vi "Intensity.vi"(8 "error in (no error)":errorcluster, 10 "Image in":T2(plugin-control), 11 "Intensity Limit":string[][](array[string])) -> (0 "error out":errorcluster, 2 "Image out":T2(plugin-control), 3 "Intensity":T1(array[cluster]))   [LabVIEW 2020]
uses:
  <vilib>/vision/NI_Vision_Development_Module.lvlib
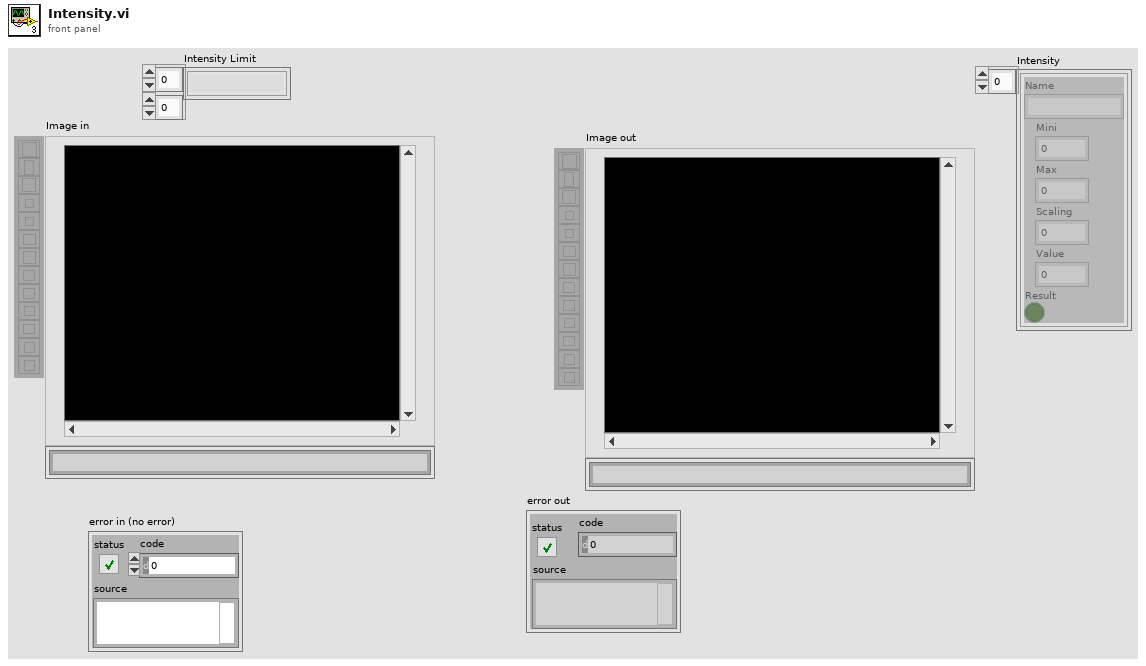
[diagram p1: front panel]
types:
  T1 = cluster{"Name":string, "Mini":dbl, "Max":dbl, "Scaling ":dbl, "Value ":dbl, "Result":bool}[]
  T2 = typedef "IMAQ Image.ctl" = refnum<image>
  T3 = cluster{"Name":string, "Mini":dbl, "Max":dbl, "Scaling ":dbl, "Value ":dbl, "Result":bool}
  T4 = cluster{"Global Rectangle":i32[], "Contours":cluster{"Contour Type":u32, "ROI Type":u32, "Points":i32[]}[]}
  T5 = cluster{"Left":i32, "Top":i32, "Right":i32, "Bottom":i32}
  T6 = typedef "IMAQ Rectangle" = cluster{"Left":i32, "Top":i32, "Right":i32, "Bottom":i32, "Rotation":dbl}
  T7 = cluster{"Mean Intensity":sgl, "Standard  Deviation":sgl, "Minimum Intensity":sgl, "Maximum Intensity":sgl}
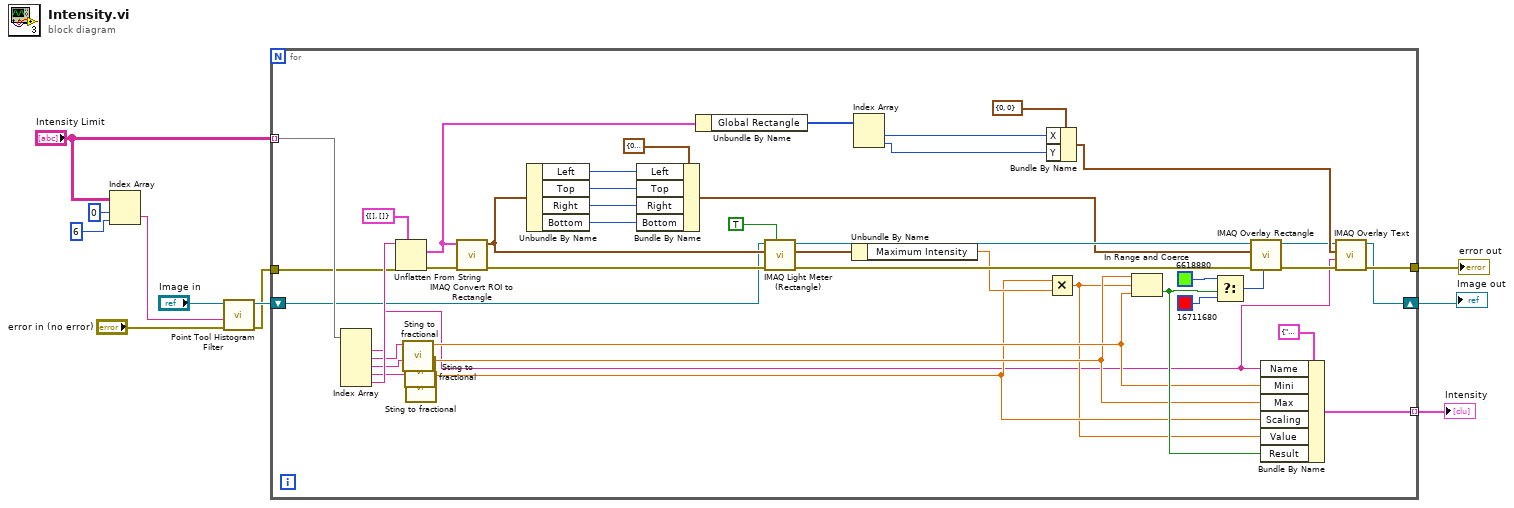
[diagram p0: block diagram]
diagram:
  n1 = Index Array(array="Intensity Limit", index (row)=0, index (col)=6 ("index (row)")) -> (element=w3:string)
  n2 = call "Point Tool Histogram Filter.vi"("error in"="error in (no error)", "Combo Box"=w3, "Image in"="Image in") -> ("error out"=w1:errorcluster, "Image out"=w8:T2)  [unwired: 7 in]
  n3 = for {
    tunnel: "Intensity Limit" -> [w42] mode=indexing
    tunnel: w1 -> [w39]
    shift-right: [w13] -> w10
    shift-left: w8 -> [w38]
    tunnel: [w33] -> w9 mode=indexing
    tunnel: [w22] -> w11
    n4 = Index Array(array=w42) -> (element #1=w12:string, element #2=w37:string, element #3=w36:string, element #4=w35:string, element #5=w41:string)  [unwired: 5 in]
    n5 = Unflatten From String(type=T4 {"Global Rectangle"=[], "Contours"=[]} ("ROI"), binary string=w41, error in (no error)=w39) -> (value=w20:T4, error out=w40:errorcluster)  [unwired: 2 in, 1 out]
    n6 = call "Sting to fractional.vi"("String"=w37) -> ("Numeric"=w27:dbl)  [unwired: 10 in]
    n7 = call "Sting to fractional.vi"("String"=w36) -> ("Numeric"=w26:dbl)  [unwired: 10 in]
    n8 = call "Sting to fractional.vi"("String"=w35) -> ("Numeric"=w25:dbl)  [unwired: 10 in]
    n9 = call "IMAQ Convert ROI to Rectangle"("error in (no error)"=w40, "ROI Descriptor"=w20) -> ("error out"=w44:errorcluster, "Rectangle"=w49:T6)  [unwired: 7 in]
    n10 = Unbundle By Name(w49) -> ("Left"=w48:i32, "Top"=w47:i32, "Right"=w46:i32, "Bottom"=w45:i32)
    n11 = Bundle By Name(cluster=T5 {"Left"=0, "Top"=0, "Right"=0, "Bottom"=0} ("Rectangle 2"), "Left"=w48, "Top"=w47, "Right"=w46, "Bottom"=w45) -> (w21:T5)
    n12 = Unbundle By Name(w20) -> ("Global Rectangle"=w19:i32[])
    n13 = call "IMAQ Light Meter (Rectangle)"("Show Search Area"=TRUE, "error in (no error)"=w44, "Rectangle"=w49, "Image"=w38) -> ("error out"=w51:errorcluster, "Gray Level Intensities"=w54:T7, "Image Out"=w52:T2)  [unwired: 3 in, 2 out]
    n14 = Unbundle By Name(w54) -> ("Maximum Intensity"=w34:sgl)
    n15 = Index Array(array=w19) -> (element #1=w17:i32, element #2=w16:i32)  [unwired: 2 in]
    n16 = Bundle By Name(cluster=cluster{"X":i32, "Y":i32} {"X"=0, "Y"=0}, "X"=w17, "Y"=w16) -> (w15:cluster{"X":i32, "Y":i32})
    n17 = Multiply(x=w25, y=w34) -> (x*y=w24:dbl)
    n18 = In Range and Coerce(upper limit=w26, x=w24, lower limit=w27) -> (In Range?=w30:bool)  [unwired: 1 out]
    n19 = Select(t=u32 6618880 ("Color"), s=w30, f=u32 16711680 ("Color")) -> (s? t:f=w29:u32)
    n20 = call "IMAQ Overlay Rectangle"("Color"=w29, "error in (no error)"=w51, "Rectangle"=w21, "Image"=w52) -> ("error out"=w23:errorcluster, "Image Out"=w14:T2)  [unwired: 6 in]
    n21 = Bundle By Name(cluster=T3 {"Name"="", "Mini"=0.0, "Max"=0.0, "Scaling "=0.0, "Value "=0.0, "Result"=FALSE}, "Name"=w12, "Mini"=w27, "Max"=w26, "Scaling"=w25, "Value"=w24, "Result"=w30) -> (w33:T3)
    n22 = call "IMAQ Overlay Text"("error in (no error)"=w23, "String"=w12, "Origin"=w15, "Image"=w14) -> ("error out"=w22:errorcluster, "Image Out"=w13:T2)  [unwired: 6 in]
  }
  "Image out" <- w10
  "error out" <- w11
  "Intensity" <- w9
